vi "flatten.vi"(8 "error in":errorcluster, 11 "test-group in":refnum<class "test-group.lvclass">) -> (0 "error out":errorcluster, 2 "flattened group":string, 3 "test-group out":refnum<class "test-group.lvclass">)   [LabVIEW 2020, in "test-group.lvclass"]
uses:
  test-group.lvclass
  test-group.lvclass/test-group.ctl
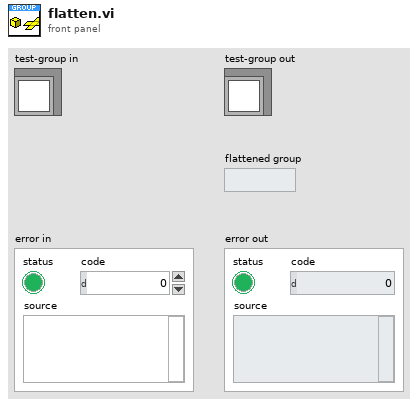
[diagram p1: front panel]
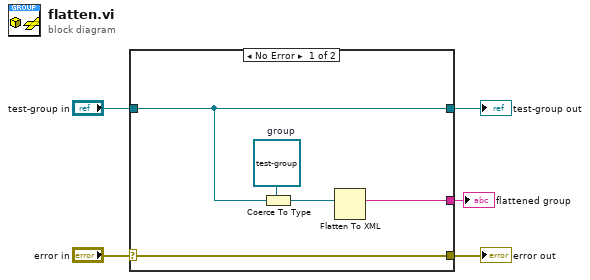
[diagram p0: block diagram]
diagram:
  n1 = case shown="No Error" "error in" {
    selector: "error in" -> [w10 w12]
    tunnel: [w10 w12] -> w4
    tunnel: [w9 w11] -> w2
    tunnel: "test-group in" -> [w9 w11]
    tunnel: [w8 _] -> w1
    frame No Error {
      w6 = refnum<class "test-group.lvclass"> refnum  # group
      n2 = Coerce To Type(0:w9, 1:w6) -> (2:w7:refnum<class "test-group.lvclass">)
      n3 = Flatten To XML(6:w7) -> (2:w8:string)
    }
    frame Error {
    }
  }
  "error out" <- w4
  "test-group out" <- w2
  "flattened group" <- w1
